vi "Client.vi"() -> ()   [LabVIEW 2020]
uses:
  Chat Window/Chat Window.lvclass
  C:/Program Files (x86)/National Instruments/LabVIEW 2020/vi.lib/ActorFramework/Actor/Actor.lvclass
  Chat Window/Chat Window.lvclass/Chat Window.ctl
  <vilib>/NI/Actors/Network Endpoint Actors/Protocols/TCP Strategy/TCP Stream Initiator/TCP Stream Initiator.lvclass
  C:/Program Files (x86)/National Instruments/LabVIEW 2020/vi.lib/NI/Actors/Network Endpoint Actors/Abstract Classes/Message Stream/Message Stream.lvclass
  <vilib>/ActorFramework/Actor/Actor.lvclass
panel:
  in  "Remote Port":u16=2001
  in  "Remote Address":string="127.0.0.1"
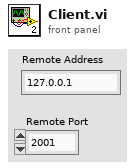
[diagram p1: front panel]
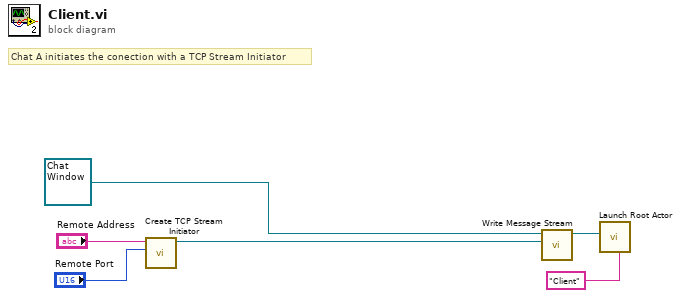
[diagram p0: block diagram]
diagram:
  # "Chat A initiates the conection with a TCP Stream Initiator"
  n1 = call <vilib>:"Create TCP Stream Initiator.vi"("Remote Port"="Remote Port", "Remote Address"="Remote Address") -> ("TCP Stream Initiator"=w1:refnum<class "TCP Stream Initiator.lvclass">)  [unwired: 9 in]
  n2 = call "Write Message Stream.vi"("Message Stream"=w1, "Chat Window in"=refnum<class "Chat Window.lvclass"> refnum) -> ("Chat Window out"=w3:refnum<class "Chat Window.lvclass">)  [unwired: 9 in]
  n3 = call <vilib>:"Launch Root Actor.vi"("Debug Alias"="Client", "Actor"=w3) -> ()  [unwired: 8 in, 2 out]
